vi "DSF.Engine.Builder.Initialize.vi"(8 "error in (no error)":errorcluster, 11 "Builder in":refnum<class "DSF.Engine.Builder.lvclass">) -> (0 "error out":errorcluster, 2 "response":T1, 3 "Builder out":refnum<class "DSF.Engine.Builder.lvclass">, 4 "VS Channels Buffer":dbl[](array[numeric]), 5 "Data Type Buffers":T3)   [LabVIEW 2016, in "DSF.Engine.lvlib" / "DSF.Engine.Builder.lvclass"]
uses:
  DSF.Engine.Builder.lvclass
  Typedefs/DSF.Engine.Typedefs.Type Buffers.ctl
  Interface/DSF.Engine.Interface.Builder.Response Data.ctl
  Interface/DSF.Engine.Interface.Builder.Response.ctl
  Interface/DSF.Engine.Interface.Builder.lvclass
  DSF.Engine.lvlib
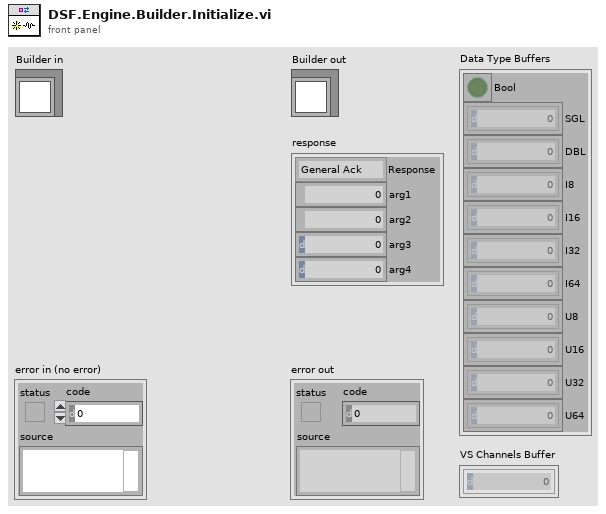
[diagram p1: front panel]
types:
  T1 = typedef "DSF.Engine.lvlib/DSF.Engine.Interface.Builder.lvclass/DSF.Engine.Interface.Builder.Response Data.ctl" = cluster{"Response":T2, "arg1":i32, "arg2":i32, "arg3":i32, "arg4":i32}
  T2 = typedef "DSF.Engine.lvlib/DSF.Engine.Interface.Builder.lvclass/DSF.Engine.Interface.Builder.Response.ctl" = enum8{"General Ack", "Initialize Complete", "Build Complete", "Parse Complete", "Shutdown Ack"}
  T3 = typedef "DSF.Engine.lvlib/DSF.Engine.Typedefs.Type Buffers.ctl" = cluster{"Bool":bool[], "SGL":sgl[], "DBL":dbl[], "I8":i8[], "I16":i16[], "I32":i32[], "I64":i64[], "U8":u8[], "U16":u16[], "U32":u32[], "U64":u64[]}
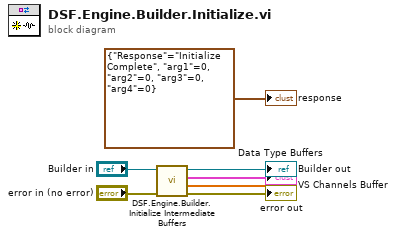
[diagram p0: block diagram]
diagram:
  n1 = call "DSF.Engine.Builder.Initialize Intermediate Buffers.vi"("error in (no error)"="error in (no error)", "Builder in"="Builder in") -> ("error out"=→"error out":errorcluster, "VS Channels Buffer"=→"VS Channels Buffer":dbl[], "Data Type Buffers"=→"Data Type Buffers":T3, "Builder out"=→"Builder out":refnum<class "DSF.Engine.Builder.lvclass">)  [unwired: 6 in]
  "response" <- T1 {"Response"=enum."Initialize Complete", "arg1"=0, "arg2"=0, "arg3"=0, "arg4"=0} ("response")
